vi "Sept16Prop.vi"() -> ()   [LabVIEW 2015]
uses:
  <vilib>/Platform/TimedLoop/XDataNode/timing_clust.ctl
  <vilib>/Platform/TimedLoop/XDataNode/nitl_modes.ctl
  <vilib>/Platform/TimedLoop/XDataNode/wakeup.ctl
  <vilib>/FPGAPlugInAG/myRIO-1900/niLvFpga_Open_myRIO-1900.vi
  <vilib>/rvi/interface/common/dynamic/niFpgaDynamicAddResources.vi
  <vilib>/Utility/file.llb/Write Delimited Spreadsheet (DBL).vi
  <vilib>/Utility/error.llb/Error Cluster From Error Code.vi
  <vilib>/rvi/errors/niLvFpgaAdjustHostInterfaceError.vi
  <vilib>/FPGAPlugInAG/Dynamic/niLvFpga_Close_Dynamic.vi
  <vilib>/rvi/interface/nirviOpenFPGA/nirviOpenFPGA.xnode
  FPGA Bitfiles/ViconProj_FPGATarget_CurrentControlle_6L7CFhOQTHY.lvbitx
  Misc/Current Controller.vi
  <vilib>/platform/TimedLoop/XDataNode/XDataNode.xnode
  <vilib>/rvi/interface/nirviReadWriteControl/nirviReadWriteControl.xnode
  <vilib>/rvi/interface/nirviCloseFPGA/nirviCloseFPGA.xnode
  <vilib>/rvi/interface/Simulation/niFpgaSimulationCallBeginRW.vi
  <vilib>/Platform/TimedLoop/XDataNode/XDNodeRunTimeDep.lvlib
  NiFpgaLv.dll
panel:
  in  "Tab Control":enum32{"Page 1"}(tab)
  out "Rotation":dbl[][](graph)
  out "Translation":dbl[][](graph)
  in  "Stop":bool
  out "x":dbl
  out "z":dbl
  out "y":dbl
  out "roll":dbl
  out "pitch":dbl
  out "yaw":dbl
  in  "Current (mA)":i32(knob)=321 scale=60.0..600.0
  out "error out":errorcluster
  out "Overflow?":bool
  in  "stop":bool
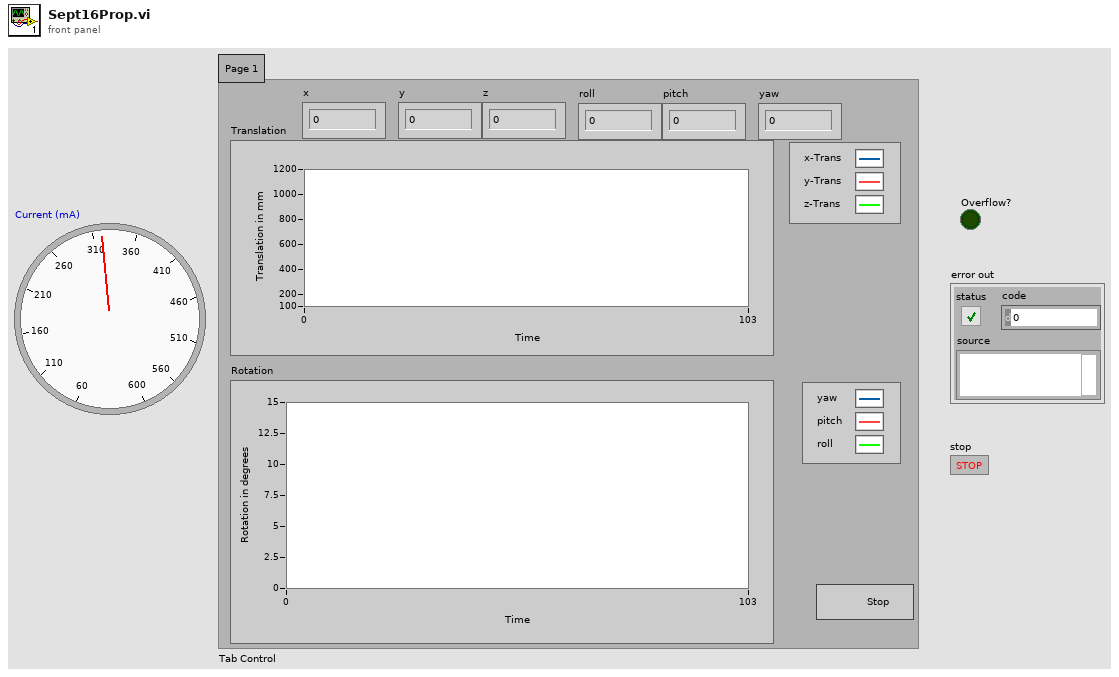
[diagram p1: front panel]
types:
  T1 = typedef "XDNodeRunTimeDep.lvlib/timing_clust.ctl" = cluster{"Expected End [f-1]":u64, "Actual End [f-1]":u64, "Finished Late? [f-1]":bool, "Expected End [i-1]":u64, "Actual End [i-1]":u64, "Finished Late? [i-1]":bool, "Expected Start [i]":u64, "Actual Start [i]":u64, "Expected Start [f]":u64, "Actual Start [f]":u64, "Source Name":string, "Structure Name":string, "Period":i64, "Deadline":i64, "Offset":i64, "Start":i64, "Priority":i32, "Timeout":i32, "Mode":T2, "Wakeup Reason":T3, "Error":errorcluster, "Source Type":string, "Secondary Source Type":string, "Global End Time":u64, "Global Start Time":u64, "Frame Duration":u64, "Iteration Duration":u64, "Assigned CPU":i32, "I/O Scan Engine Mode":u32}
  T2 = typedef "XDNodeRunTimeDep.lvlib/nitl_modes.ctl" = enum32{"No Change", "Process missed periods, maintain original phase", "Discard missed periods, maintain original phase", "Process missed periods, ignore original phase", "Discard missed periods, ignore original phase"}
  T3 = typedef "XDNodeRunTimeDep.lvlib/wakeup.ctl" = enum32{"Normal", "Aborted", "Asynchronous wakeup", "Timing source error", "Timed loop error", "Timeout"}
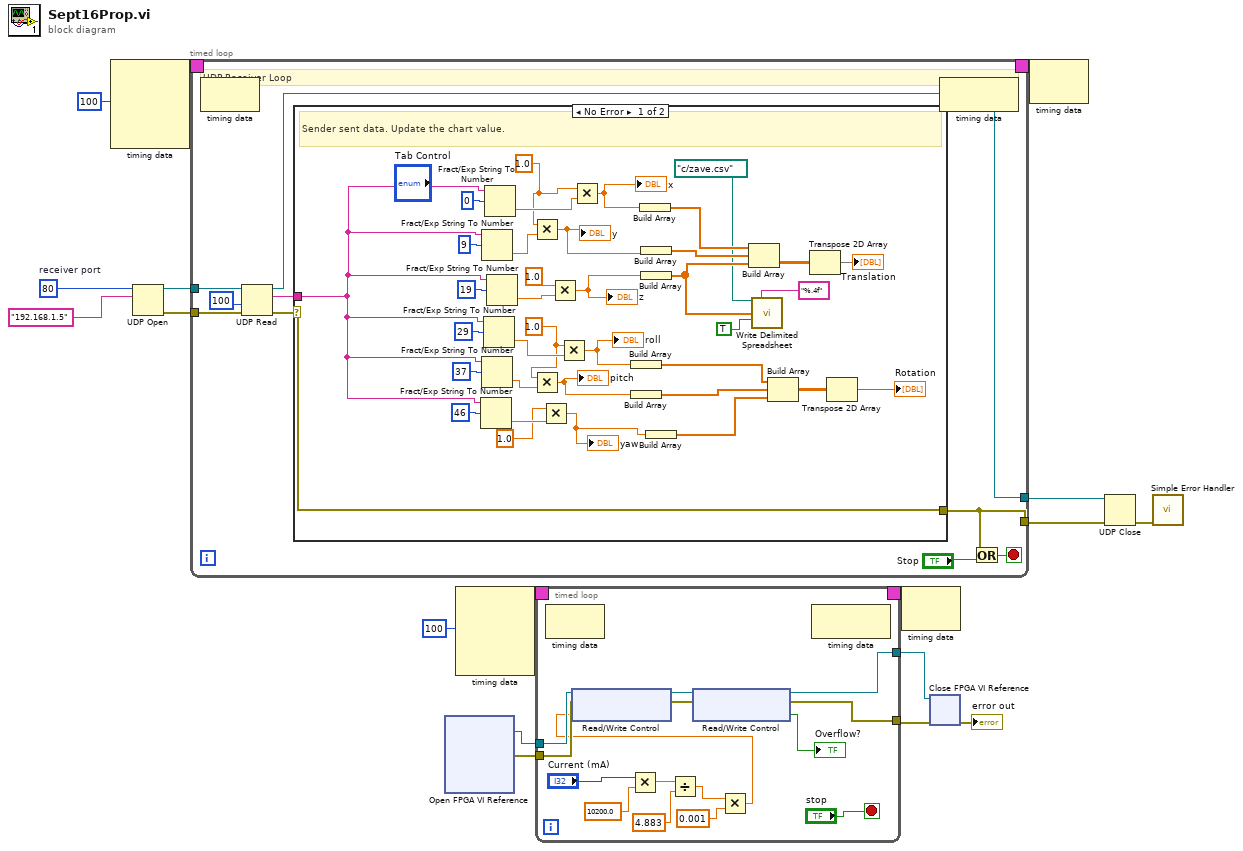
[diagram p0: block diagram]
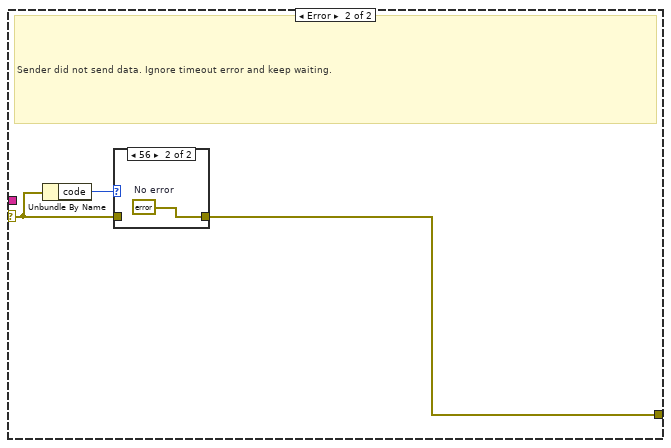
[diagram p2: hidden frame]
diagram:
  w8 = u16 80  # receiver port
  n1 = node-c288(i64 100 ("Period")) -> (w6:T1)  [unwired: 3 in]
  n2 = UDP Open(10:"192.168.1.5" ("service name"), 11:w8) -> (port=w9:refnum<k16>, 0:w10:errorcluster)  [unwired: 3 in, 1 out]
  n3 = timed-loop {
    tunnel: w9 -> [w27]
    tunnel: [w19] -> w13
    tunnel: w10 -> [w24]
    tunnel: [w20] -> w11
    timing: w6 -> [_]
    timing-out: [_] -> w5
    stop <- w25 stop-if-true
    # "UDP Receiver Loop"
    n4 = node-c288() -> ()  [unwired: 1 in, 1 out]
    n5 = UDP Read(connection ID=w27, timeout ms (25000)=100, 8:w24) -> (data out=w22:string, error out=w21:errorcluster, 3:w19:refnum<k16>)  [unwired: 3 out]
    n6 = case shown="No Error" w21 {
      selector: w21 -> [w66 w68]
      tunnel: w22 -> [w36 _]
      tunnel: [w66 w67] -> w20
      frame No Error {
        w42 = 1.0 ("x")
        w35 = 1.0 ("y")
        # "Sender sent data. Update the chart value."
        n7 = Fract/Exp String To Number(string=w36, offset=46) -> (number=w39:dbl)  [unwired: 2 in, 1 out]
        n8 = Fract/Exp String To Number(string=w36, offset=9) -> (number=w46:dbl)  [unwired: 2 in, 1 out]
        n9 = Fract/Exp String To Number(string=w36, offset=37) -> (number=w41:dbl)  [unwired: 2 in, 1 out]
        n10 = Fract/Exp String To Number(string=w36, offset=29) -> (number=w44:dbl)  [unwired: 2 in, 1 out]
        n11 = Fract/Exp String To Number(string=w36, offset=0) -> (number=w49:dbl)  [unwired: 2 in, 1 out]
        n12 = Fract/Exp String To Number(string=w36, offset=19) -> (number=w48:dbl)  [unwired: 2 in, 1 out]
        n13 = Multiply(x=w35, y=w46) -> (x*y=w45:dbl)
        "y" <- w45
        n14 = Multiply(x=w42, y=w41) -> (x*y=w40:dbl)
        "pitch" <- w40
        n15 = Multiply(x=1.0, y=w39) -> (x*y=w37:dbl)
        "yaw" <- w37
        n16 = Multiply(x=1.0, y=w48) -> (x*y=w34:dbl)
        "z" <- w34
        n17 = Multiply(x=w42, y=w44) -> (x*y=w43:dbl)
        "roll" <- w43
        n18 = Multiply(x=w35, y=w49) -> (x*y=w50:dbl)
        "x" <- w50
        n19 = Build Array(w43) -> (w53:dbl[])
        n20 = Build Array(w40) -> (w54:dbl[])
        n21 = Build Array(w50) -> (w57:dbl[])
        n22 = Build Array(w45) -> (w56:dbl[])
        n23 = Build Array(w34) -> (w33:dbl[])
        n24 = Build Array(w37) -> (w55:dbl[])
        n25 = Build Array(w57, w56, w33) -> (w62:dbl[][])
        n26 = call-poly <vilib>:"Write Delimited Spreadsheet.vi"("file path (dialog if empty)"=path "c:/zave.csv", "format (%.3f)"="%.4f", "1D data"=w33, "append to file? (F)"=TRUE) -> ()  [unwired: 10 in, 2 out]
        n27 = Build Array(w53, w54, w55) -> (w52:dbl[][])
        n28 = Transpose 2D Array(2D array=w62) -> (transposed array=→"Translation":dbl[][])
        n29 = Transpose 2D Array(2D array=w52) -> (transposed array=→"Rotation":dbl[][])
      }
      frame Error {
        # "Sender did not send data. Ignore timeout error and keep waiting."
        n30 = Unbundle By Name(w68) -> ("code"=w69:i32)
        n31 = case shown="56" w69 {
          tunnel: w68 -> [w70 _]
          tunnel: [w70 w71] -> w67
          frame Default {
          }
          frame 56 {
            w71 = errorcluster {"status"=FALSE, "code"=0, "source"=""}  # No error
          }
        }
      }
    }
    n32 = node-c288() -> ()  [unwired: 1 in, 1 out]
    n33 = Or(x=w20, y="Stop") -> (x .or. y?=w25:bool)
  }
  n34 = xnode "Open FPGA VI Reference"() -> ("FPGA VI Reference Out"=w18:refnum<k20>, "error out"=w17:errorcluster)  [unwired: 2 in]
  n35 = node-c288(i64 100 ("Period")) -> (w4:T1)  [unwired: 3 in]
  n36 = timed-loop {
    tunnel: w18 -> [w85]
    tunnel: w17 -> [w84]
    tunnel: [w81] -> w16
    tunnel: [w73] -> w15
    timing: w4 -> [_]
    timing-out: [_] -> w3
    stop <- "stop" stop-if-true
    n37 = node-c288() -> ()  [unwired: 1 in, 1 out]
    n38 = Multiply(x="Current (mA)", y=10200.0) -> (x*y=w78:dbl)
    n39 = Divide(x=w78, y=4.883) -> (x/y=w75:dbl)
    n40 = Multiply(x=w75, y=0.001) -> (x*y=w74:dbl)
    n41 = xnode "Read/Write Control"("FPGA VI Reference In"=w85, "error in"=w84, "DAC Inlet Valve"=w74) -> ("FPGA VI Reference Out"=w83:refnum<k20>, "error out"=w82:errorcluster)
    n42 = xnode "Read/Write Control"("FPGA VI Reference In"=w83, "error in"=w82) -> ("FPGA VI Reference Out"=w81:refnum<k20>, "error out"=w73:errorcluster, "Inlet Overflow?"=→"Overflow?":bool)
    n43 = node-c288() -> ()  [unwired: 1 in, 1 out]
  }
  n44 = node-c288(w3) -> ()  [unwired: 1 out]
  n45 = xnode "Close FPGA VI Reference"("FPGA VI Reference In"=w16, "error in"=w15) -> ("error out"=→"error out":errorcluster)
  n46 = node-c288(w5) -> ()  [unwired: 1 out]
  n47 = UDP Close(connection ID=w13, 8:w11) -> (error out=w12:errorcluster)  [unwired: 1 out]
  n48 = call <vilib>:"Simple Error Handler.vi"("error in (no error)"=w12) -> ()  [unwired: 1 in, 8 out]
